vi "Climber_Sequencer.vi"() -> (0 "Outer_Arm_Elevator":dbl, 1 "Inner_Arm_Pivot":dbl, 2 "Outer_Arm_Pivot":dbl)   [LabVIEW 2020]
panel:
  in  "reset":bool
  in  "inner_arm_rotation":dbl
  in  "outer_arm_rotation":dbl
  in  "d1":dbl
  in  "outer_arm_position":dbl
  out "step":i32
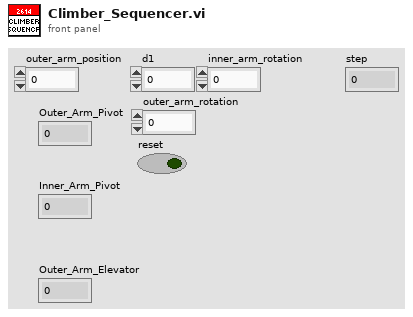
[diagram p1: front panel]
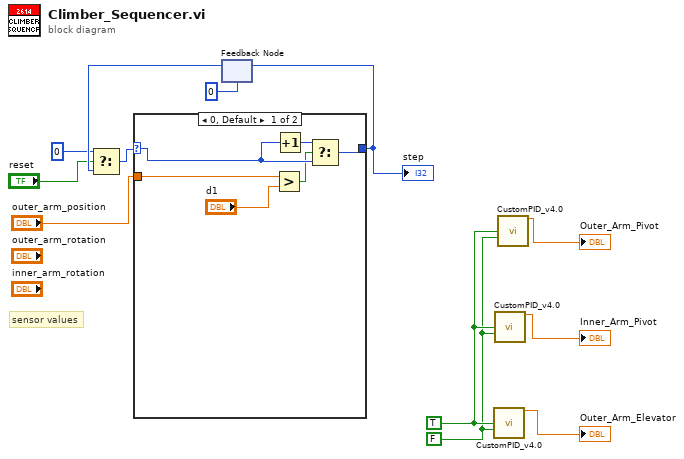
[diagram p0: block diagram]
diagram:
  w1 = FALSE ("Reset on Goal Change ?")
  w2 = TRUE ("Reset on Goal Change ?")
  # "sensor values"
  n1 = feedback #1(0) -> (w9:i32)
  n2 = Select(t=0, s="reset", f=w9) -> (s? t:f=w10:i32)
  n3 = case shown="0, Default" w10 {
    selector: w10 -> [w17 _]
    tunnel: [w18 _] -> w12
    tunnel: "outer_arm_position" -> [w13 _]
    frame 0, Default {
      n4 = Greater?(x=w13, y="d1") -> (0:w15:bool)
      n5 = Increment(x=w17) -> (x+1=w16:i32)
      n6 = Select(t=w16, s=w15, f=w17) -> (s? t:f=w18:i32)
    }
    frame 1 {
    }
  }
  "step" <- w12
  n7 = feedback-in #1(w12) -> ()
  n8 = call "CustomPID_v4.0.vi"("Reset on Goal Change ?"=w2, "Use Custom Error Calculation ?"=w1) -> ("Command"=→"Outer_Arm_Elevator":dbl)  [unwired: 10 in, 3 out]
  n9 = call "CustomPID_v4.0.vi"("Reset on Goal Change ?"=w2, "Use Custom Error Calculation ?"=w1) -> ("Command"=→"Inner_Arm_Pivot":dbl)  [unwired: 10 in, 3 out]
  n10 = call "CustomPID_v4.0.vi"("Reset on Goal Change ?"=w2, "Use Custom Error Calculation ?"=w1) -> ("Command"=→"Outer_Arm_Pivot":dbl)  [unwired: 10 in, 3 out]
